vi "send_pipette_to_AnalysisObj.vi"(0 "SessionID":string, 5 "pipette_name":string, 7 "dilution factor":dbl, 9 "pipette counter":u32, 11 "error in (no error)":errorcluster, 12 "number of shots":u32) -> (15 "error out":errorcluster)   [LabVIEW 2018]
doc: "sendds the data to the AnalysisSession (SessionID) and stores them in the PipetteDataArray"
uses:
  global variables.vi
  Classes/StatusLog/StatusLog.lvclass
  Classes/Analysis/Analysis.lvclass
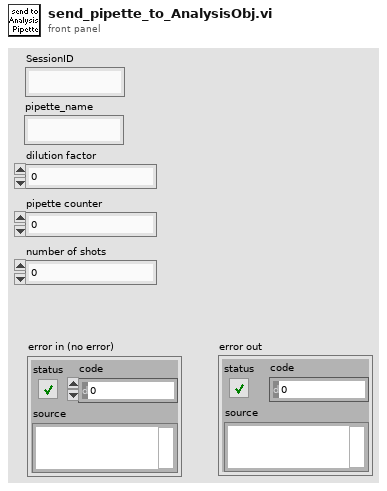
[diagram p1: front panel]
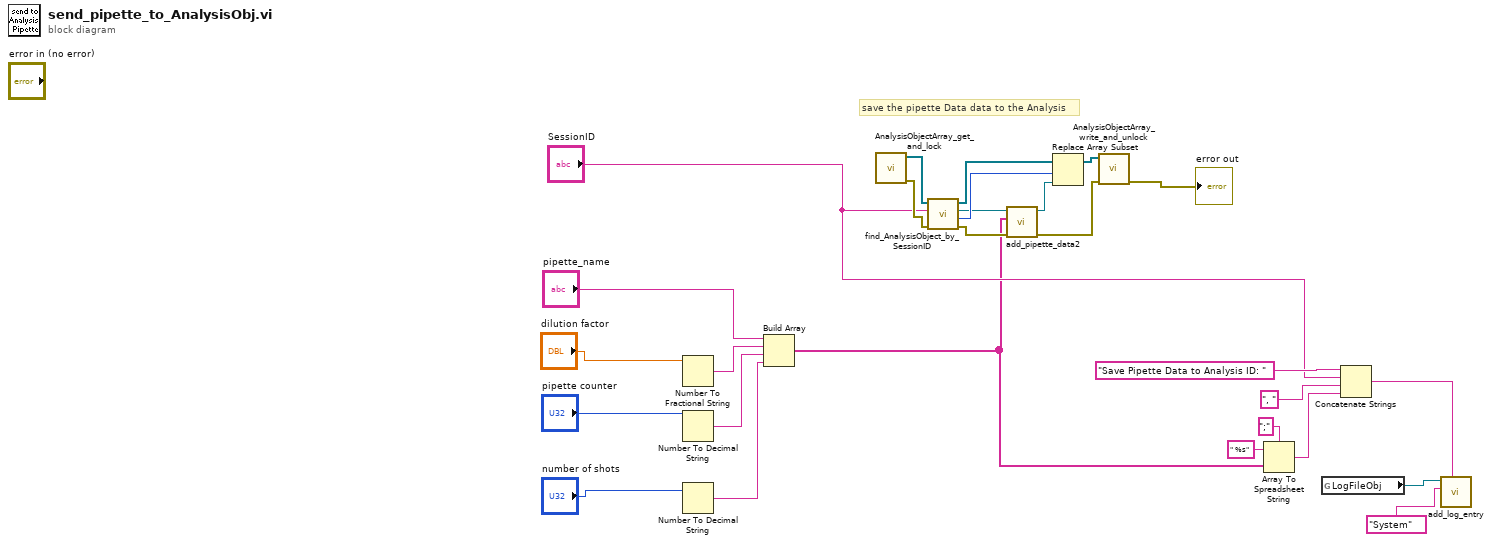
[diagram p0: block diagram]
diagram:
  # "save the pipette Data data to the Analysis"
  n1 = Number To Fractional String(number="dilution factor") -> (F-format string=w17:string)  [unwired: 3 in]
  n2 = Number To Decimal String(number="pipette counter") -> (decimal integer string=w13:string)  [unwired: 1 in]
  n3 = Number To Decimal String(number="number of shots") -> (decimal integer string=w11:string)  [unwired: 1 in]
  n4 = Build Array("pipette_name", w17, w13, w11) -> (w5:string[])
  n5 = call "AnalysisObjectArray_get_and_lock.vi"() -> ("error out"=w23:errorcluster, "AnalysisObjects"=w22:refnum<class "Analysis.lvclass">[])  [unwired: 10 in]
  n6 = call "find_AnalysisObject_by_SessionID.vi"("error in (no error)"=w23, "SessionID"="SessionID", "AnalysisObjects in"=w22) -> ("error out"=w20:errorcluster, "index of found"=w25:i32, "found AnalyisObject"=w21:refnum<class "Analysis.lvclass">, "AnalysisObjects out"=w24:refnum<class "Analysis.lvclass">[])  [unwired: 5 in]
  n7 = call-dynamic "add_pipette_data2.vi"("error in (no error)"=w20, "pipette data"=w5, "Analysis in"=w21) -> ("error out"=w19:errorcluster, "Analysis out"=w18:refnum<class "Analysis.lvclass">)  [unwired: 7 in]
  n8 = Replace Array Subset(array=w24, new element=w18, index=w25) -> (w26:refnum<class "Analysis.lvclass">[])
  n9 = call "AnalysisObjectArray_write_and_unlock.vi"("error in (no error)"=w19, "AnalysisObjects"=w26) -> ("error out"=→"error out":errorcluster)  [unwired: 9 in]
  n10 = Array To Spreadsheet String(delimiter (Tab)=";", array=w5, 3:" %s" ("format string")) -> (spreadsheet string=w4:string)
  n11 = global read "global variables.vi" "LogFileObj"() -> (w10:refnum<class "StatusLog.lvclass">)
  n12 = Concatenate Strings("Save Pipette Data to Analysis ID: ", "SessionID", ", " ("string"), w4) -> (w3:string)
  n13 = call-dynamic "add_log_entry.vi"("new entry"=w3, "log identifiers"="System", "StatusLog in"=w10) -> ()  [unwired: 5 in, 2 out]
